vi "file IO main.vi"(11 "fileIO":T1) -> ()   [LabVIEW 2018]
uses:
  type defs/file IO data.ctl
  type defs/channelControl.ctl
  RT/Type Defs/channelScalingTypes.ctl
  RT/Type Defs/scalingMethods.ctl
  ICL-LabVIEW_General/data channels/parent class/Data Channel.lvclass
  ICL-LabVIEW_General/data channels/parent class/channel type.ctl
  ICL-LabVIEW_General/data channels/parent class/Data Channel.lvclass/Data Channel.ctl
  supporting VIs/polymorphic VIs/de-queue for file IO.vi
  supporting VIs/polymorphic VIs/enqueue for user interface.vi
  supporting VIs/polymorphic VIs/enqueue for message handler.vi
  supporting VIs/polymorphic VIs/release file IO queue.vi
  ICL-LabVIEW_General/data channels/data channels.lvlib
panel:
  out "logging":bool
  out "current logfile":path
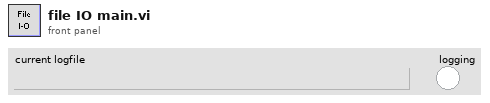
[diagram p1: front panel]
types:
  T1 = typedef "file IO data.ctl" = cluster{"params":cluster{"startFolder":path, "channelConfigPath":path}, "vars":cluster{"channelConfig ":T2[], "writing":cluster{"streaming":bool, "fixedLength":bool, "pointCount":u32, "timeZero":dbl, "pointsWritten":u32, "dataRate":u16}, "channelCount":u16, "fileTarget":cluster{"Save folder":path, "Target filename":string, "file ref":refnum<file>, "pulsatorSpeed":string, "motorSpeed":string, "valvePosition":string, "torqueFilter":bool, "pulsatorRunning":bool, "motorRunning":bool}, "channels":refnum<class "Data Channel.lvclass">[]}}
  T2 = typedef "channelControl.ctl" = cluster{"index":u16, "active":bool, "channelType":T3, "module":u16, "terminal":u16, "channelName":string, "scalingMethod":T4, "scalingParameters":dbl[], "scaledUnits":string, "tempOffset":dbl}
  T3 = typedef "channelScalingTypes.ctl" = enum16{"calculation", "measurement", "scanivalve", "output", "digital"}
  T4 = typedef "scalingMethods.ctl" = enum16{"none", "linear", "thermocouple", "polynomial", "encoder", "RTD"}
  T5 = typedef "Queues.ctl" = cluster{"messageHandler":refnum<queue>, "comms":refnum<queue>, "dataStream":refnum<queue>, "dataProcessor":refnum<queue>, "fileIO":refnum<queue>, "userInterface":refnum<queue>, "errors":refnum<queue>, "customCompressor":refnum<queue>}
  T6 = typedef "data channels.lvlib/Data Channel.lvclass/channel type.ctl" = enum16{"acquisition", "output", "other"}
  T7 = cluster{"total":cluster{"channels":u16, "FIFO":u16, "Scanivalve":u16, "Remote":u16, "Calculated":u16}, "active":cluster{"channels":u16, "FIFO":u16, "Scanivalve":u16, "Remote":u16, "Calculated":u16}}
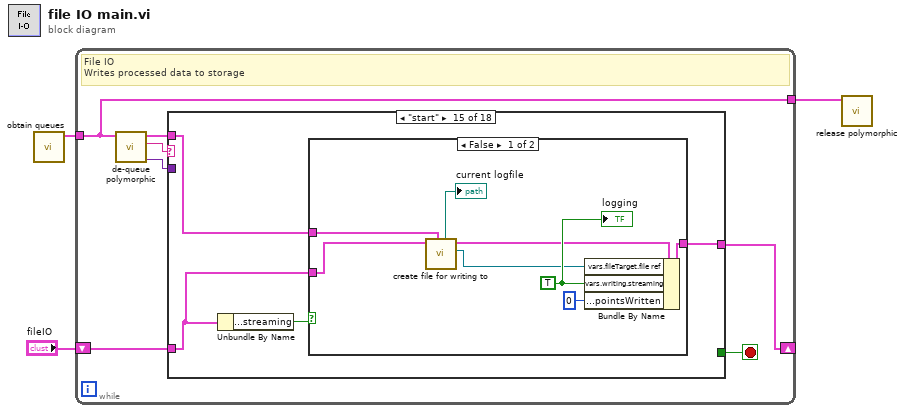
[diagram p0: block diagram]
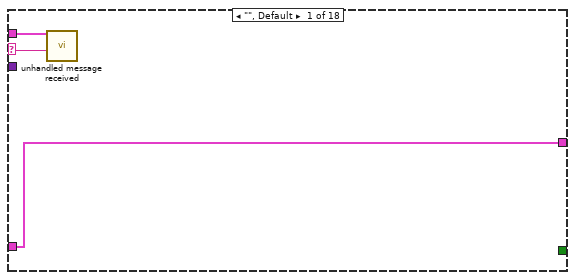
[diagram p2: hidden frame]
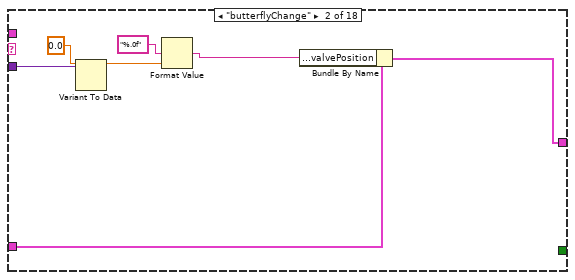
[diagram p3: hidden frame]
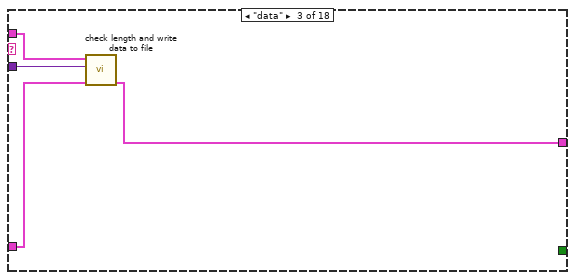
[diagram p4: hidden frame]
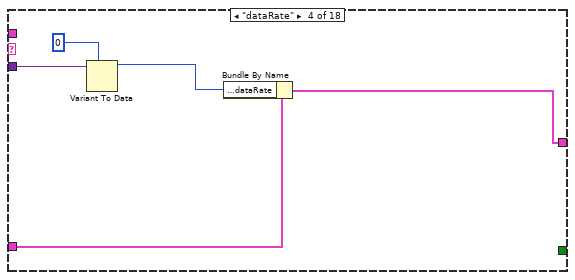
[diagram p5: hidden frame]
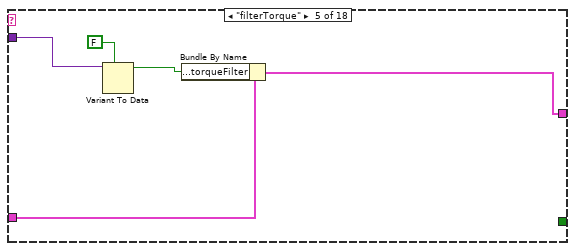
[diagram p6: hidden frame]
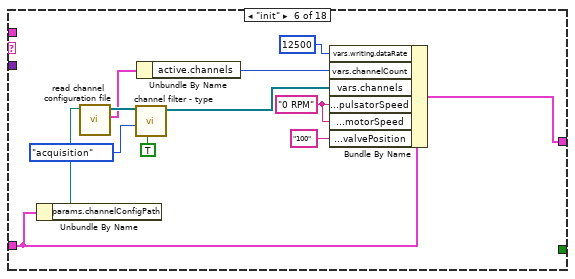
[diagram p7: hidden frame]
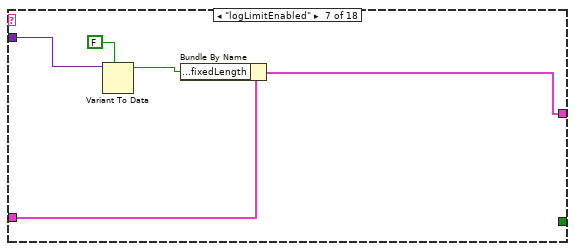
[diagram p8: hidden frame]
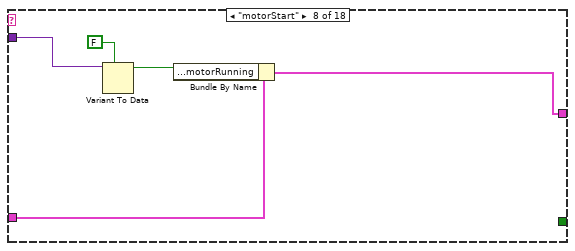
[diagram p9: hidden frame]
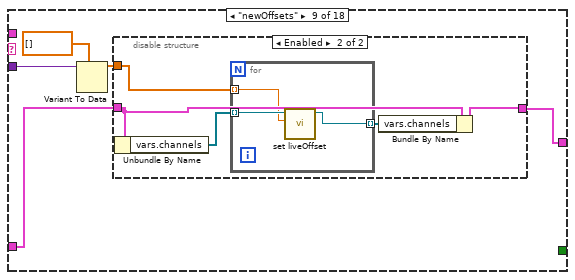
[diagram p10: hidden frame]
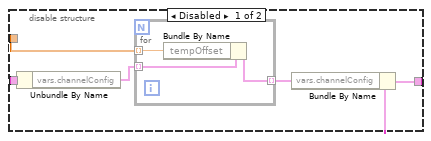
[diagram p11: hidden frame]
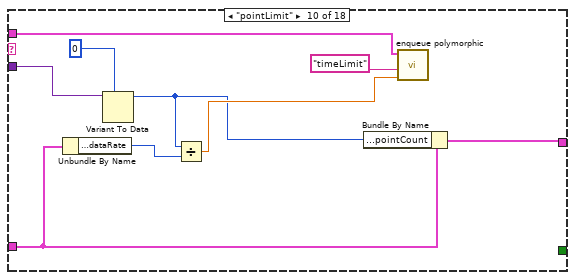
[diagram p12: hidden frame]
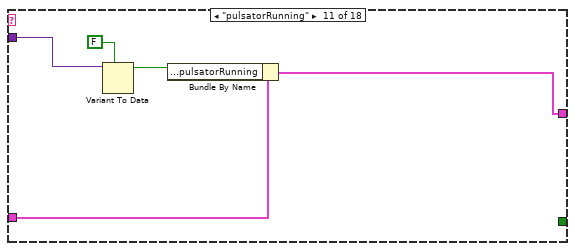
[diagram p13: hidden frame]
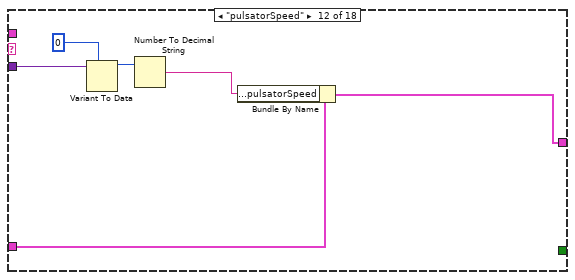
[diagram p14: hidden frame]
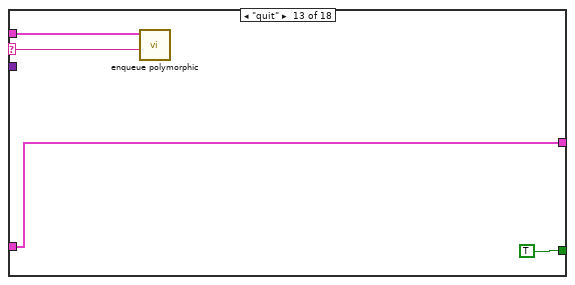
[diagram p15: hidden frame]
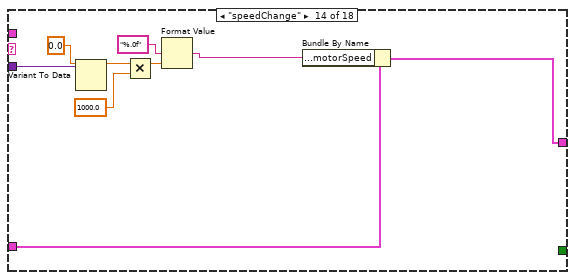
[diagram p16: hidden frame]
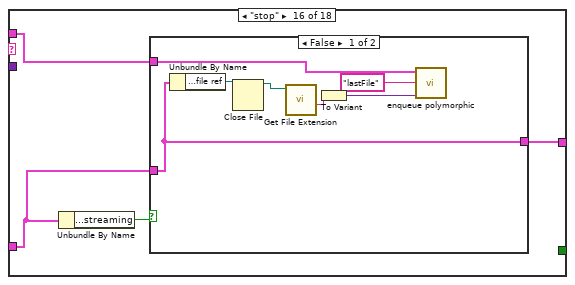
[diagram p18: hidden frame]
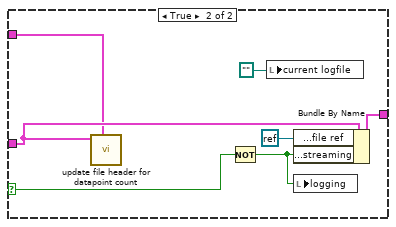
[diagram p19: hidden frame]
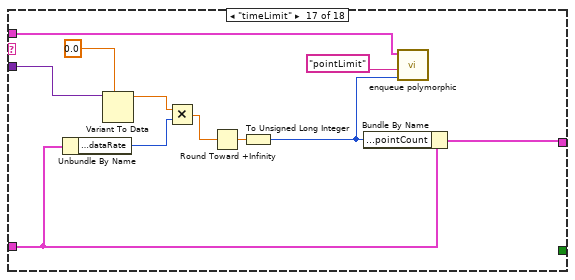
[diagram p20: hidden frame]
diagram:
  n1 = call "obtain queues.vi"() -> ("queues"=w2:T5)  [unwired: 11 in]
  n2 = while {
    tunnel: w2 -> [w6]
    tunnel: [w6] -> w1
    shift-right: [w4] -> _
    shift-left: "fileIO" -> [w5]
    stop <- w7 stop-if-true
    # "File IO\nWrites processed data to storage"
    n3 = call-poly "de-queue polymorphic.vi"("Queues"=w6) -> ("data"=w8:variant, "message"=w9:string, "Queues out"=w10:T5)  [unwired: 8 in]
    n4 = case shown="\"start\"" w9 {
      selector: w9 -> [w11 _ _ _ _ _ _ _ _ _ _ _ w99 _ _ _ _ _]
      tunnel: w10 -> [w12 _ w21 _ _ _ _ _ _ w82 _ _ w100 _ w111 w124 w144 w157]
      tunnel: w8 -> [_ w18 w24 w27 w30 _ w47 w52 w61 w85 w87 w95 _ w108 _ _ w151 _]
      tunnel: [_ _ _ _ _ _ _ _ _ _ _ _ TRUE _ _ _ _ _] -> w7
      tunnel: w5 -> [w13 w20 w22 w29 w34 w46 w51 w56 w59 w83 w91 w97 w98 w110 w113 w126 w149 w158]
      tunnel: [w13 w19 w23 w28 w33 w45 w50 w55 w58 w86 w90 w96 w98 w109 w112 w125 w152 w158] -> w4
      frame "", Default {
        n5 = call "unhandled message received.vi"("unhandledMessage"=w11, "queues"=w12) -> ()  [unwired: 10 in]
      }
      frame "butterflyChange" {
        n6 = Variant To Data(type=0.0 ("vars.writing.dataRate"), Variant=w18) -> (data=w15:dbl)  [unwired: 1 in, 1 out]
        n7 = Format Value(format string="%.0f", value (0)=w15) -> (output string=w16:string)  [unwired: 1 in]
        n8 = Bundle By Name(cluster=w20, "vars.fileTarget.valvePosition"=w16) -> (w19:T1)
      }
      frame "data" {
        n9 = call "check length and write data to file.vi"("fileIO"=w22, "data"=w24, "queues"=w21) -> ("output cluster"=w23:T1)  [unwired: 8 in]
      }
      frame "dataRate" {
        n10 = Variant To Data(type=u16 0 ("vars.writing.dataRate"), Variant=w27) -> (data=w25:u16)  [unwired: 1 in, 1 out]
        n11 = Bundle By Name(cluster=w29, "vars.writing.dataRate"=w25) -> (w28:T1)
      }
      frame "filterTorque" {
        n12 = Variant To Data(type=FALSE ("vars.writing.fixedLength"), Variant=w30) -> (data=w31:bool)  [unwired: 1 in, 1 out]
        n13 = Bundle By Name(cluster=w34, "vars.fileTarget.torqueFilter"=w31) -> (w33:T1)
      }
      frame "init" {
        w43 = "0 RPM" ("vars.fileTarget.pulsatorSpeed")
        n14 = Unbundle By Name(w46) -> ("params.channelConfigPath"=w41:path)
        n15 = call "read channel configuration file.vi"("config file"=w41) -> ("counts"=w38:T7, "channelsArray"=w40:refnum<class "Data Channel.lvclass">[])  [unwired: 8 in, 1 out]
        n16 = call "channel filter - type.vi"("activeOnly (F)"=TRUE, "channelType"=channel_type."acquisition", "channels"=w40) -> ("filteredChannels"=w36:refnum<class "Data Channel.lvclass">[])  [unwired: 6 in, 2 out]
        n17 = Unbundle By Name(w38) -> ("active.channels"=w37:u16)
        n18 = Bundle By Name(cluster=w46, "vars.writing.dataRate"=u16 12500, "vars.channelCount"=w37, "vars.channels"=w36, "vars.fileTarget.pulsatorSpeed"=w43, "vars.fileTarget.motorSpeed"=w43, "vars.fileTarget.valvePosition"="100") -> (w45:T1)
      }
      frame "logLimitEnabled" {
        n19 = Variant To Data(type=FALSE ("vars.writing.fixedLength"), Variant=w47) -> (data=w48:bool)  [unwired: 1 in, 1 out]
        n20 = Bundle By Name(cluster=w51, "vars.writing.fixedLength"=w48) -> (w50:T1)
      }
      frame "motorStart" {
        n21 = Variant To Data(type=FALSE ("vars.writing.fixedLength"), Variant=w52) -> (data=w53:bool)  [unwired: 1 in, 1 out]
        n22 = Bundle By Name(cluster=w56, "vars.fileTarget.motorRunning"=w53) -> (w55:T1)
      }
      frame "newOffsets" {
        n23 = Variant To Data(type=dbl[] [], Variant=w61) -> (data=w57:dbl[])  [unwired: 1 in, 1 out]
        n24 = disable-structure shown="Enabled" {
          disable-tunnel: w59 -> [w66 w74]
          disable-tunnel: [w65 w73] -> w58
          disable-tunnel: w57 -> [w62 w71]
          frame Disabled {
            n25 = Unbundle By Name(w66) -> ("vars.channelConfig"=w63:T2[])
            n26 = for {
              tunnel: [w68] -> w64 mode=indexing
              tunnel: w63 -> [w69] mode=indexing
              tunnel: w62 -> [w67] mode=indexing
              n27 = Bundle By Name(cluster=w69, "tempOffset"=w67) -> (w68:T2)
            }
            n28 = Bundle By Name(cluster=w66, "vars.channelConfig"=w64) -> (w65:T1)
          }
          frame Enabled {
            n29 = Unbundle By Name(w74) -> ("vars.channels"=w72:refnum<class "Data Channel.lvclass">[])
            n30 = for {
              tunnel: w72 -> [w77] mode=indexing
              tunnel: w71 -> [w76] mode=indexing
              tunnel: [w75] -> w70 mode=indexing
              n31 = call "set liveOffset.vi"("liveOffset"=w76, "Data Channel in"=w77) -> ("Data Channel out"=w75:refnum<class "Data Channel.lvclass">)  [unwired: 9 in]
            }
            n32 = Bundle By Name(cluster=w74, "vars.channels"=w70) -> (w73:T1)
          }
        }
      }
      frame "pointLimit" {
        n33 = Unbundle By Name(w83) -> ("vars.writing.dataRate"=w78:u16)
        n34 = Variant To Data(type=u32 0, Variant=w85) -> (data=w79:u32)  [unwired: 1 in, 1 out]
        n35 = Divide(x=w79, y=w78) -> (x/y=w80:dbl)
        n36 = Bundle By Name(cluster=w83, "vars.writing.pointCount"=w79) -> (w86:T1)
        n37 = call-poly "enqueue polymorphic.vi"("data"=w80, "message"="timeLimit", "Queues"=w82) -> ()  [unwired: 8 in, 1 out]
      }
      frame "pulsatorRunning" {
        n38 = Variant To Data(type=FALSE ("vars.writing.fixedLength"), Variant=w87) -> (data=w88:bool)  [unwired: 1 in, 1 out]
        n39 = Bundle By Name(cluster=w91, "vars.fileTarget.pulsatorRunning"=w88) -> (w90:T1)
      }
      frame "pulsatorSpeed" {
        n40 = Variant To Data(type=0 ("vars.writing.dataRate"), Variant=w95) -> (data=w93:i32)  [unwired: 1 in, 1 out]
        n41 = Number To Decimal String(number=w93) -> (decimal integer string=w92:string)  [unwired: 1 in]
        n42 = Bundle By Name(cluster=w97, "vars.fileTarget.pulsatorSpeed"=w92) -> (w96:T1)
      }
      frame "quit" {
        n43 = call-poly "enqueue polymorphic.vi"("message"=w99, "Queues"=w100) -> ()  [unwired: 9 in, 1 out]
      }
      frame "speedChange" {
        n44 = Variant To Data(type=0.0 ("vars.writing.dataRate"), Variant=w108) -> (data=w105:dbl)  [unwired: 1 in, 1 out]
        n45 = Multiply(x=w105, y=1000.0) -> (x*y=w103:dbl)
        n46 = Format Value(format string="%.0f", value (0)=w103) -> (output string=w106:string)  [unwired: 1 in]
        n47 = Bundle By Name(cluster=w110, "vars.fileTarget.motorSpeed"=w106) -> (w109:T1)
      }
      frame "start" {
        n48 = Unbundle By Name(w113) -> ("vars.writing.streaming"=w114:bool)
        n49 = case shown="False" w114 {
          tunnel: w113 -> [w122 w123]
          tunnel: [w121 w123] -> w112
          tunnel: w111 -> [w115 _]
          frame False {
            w120 = TRUE ("vars.streaming")
            n50 = call "create file for writing to.vi"("Queues"=w115, "fileIO"=w122) -> ("Byte Stream File out"=w118:refnum<file>, "fileIO out"=w119:T1, "target filename"=→"current logfile":path)  [unwired: 7 in]
            n51 = Bundle By Name(cluster=w119, "vars.fileTarget.file ref"=w118, "vars.writing.streaming"=w120, "vars.writing.pointsWritten"=u32 0) -> (w121:T1)
            "logging" <- w120
          }
          frame True {
          }
        }
      }
      frame "stop" {
        n52 = Unbundle By Name(w126) -> ("vars.writing.streaming"=w127:bool)
        n53 = case shown="False" w127 {
          selector: w127 -> [_ w138]
          tunnel: w126 -> [w134 w141]
          tunnel: [w134 w140] -> w125
          tunnel: w124 -> [w132 w135]
          frame False {
            n54 = Unbundle By Name(w134) -> ("vars.fileTarget.file ref"=w133:refnum<file>)
            n55 = Close File(refnum=w133) -> (path=w130:path)  [unwired: 1 in, 1 out]
            n56 = call <vilib>:"Get File Extension.vi"("file"=w130) -> ("filename without extension"=w129:string)  [unwired: 6 in, 4 out]
            n57 = To Variant(anything=w129) -> (Variant=w128:variant)
            n58 = call-poly "enqueue polymorphic.vi"("data"=w128, "message"="lastFile", "Queues"=w132) -> ()  [unwired: 8 in, 1 out]
          }
          frame True {
            n59 = call "update file header for datapoint count.vi"("Queues"=w135, "fileIO"=w141) -> ()  [unwired: 10 in]
            n60 = Not(x=w138) -> (.not. x?=w137:bool)
            n61 = local write "current logfile"(path "") -> ()
            n62 = Bundle By Name(cluster=w141, "vars.fileTarget.file ref"=refnum<k0> refnum, "vars.writing.streaming"=w137) -> (w140:T1)
            n63 = local write "logging"(w137) -> ()
          }
        }
      }
      frame "timeLimit" {
        n64 = Unbundle By Name(w149) -> ("vars.writing.dataRate"=w148:u16)
        n65 = Variant To Data(type=0.0, Variant=w151) -> (data=w147:dbl)  [unwired: 1 in, 1 out]
        n66 = Multiply(x=w147, y=w148) -> (x*y=w146:dbl)
        n67 = Round Toward +Infinity(x=w146) -> (ceil(x): smallest int >= x=w145:dbl)
        n68 = To Unsigned Long Integer(number=w145) -> (unsigned 32bit integer=w143:u32)
        n69 = Bundle By Name(cluster=w149, "vars.writing.pointCount"=w143) -> (w152:T1)
        n70 = call-poly "enqueue polymorphic.vi"("data"=w143, "message"="pointLimit", "Queues"=w144) -> ()  [unwired: 8 in, 1 out]
      }
      frame "timeLimitUpdate" {
        n71 = Unbundle By Name(w158) -> ("vars.writing.pointCount"=w153:u32, "vars.writing.dataRate"=w154:u16)
        n72 = Divide(x=w153, y=w154) -> (x/y=w155:dbl)
        n73 = call-poly "enqueue polymorphic.vi"("data"=w155, "message"="timeLimit", "Queues"=w157) -> ()  [unwired: 8 in, 1 out]
      }
    }
  }
  n74 = call-poly "release polymorphic.vi"("Queues"=w1) -> ()  [unwired: 11 in]
